vi "Close.vi"(8 "error in (no error)":errorcluster, 11 "SS P100 Settings":T1) -> (0 "error out":errorcluster, 3 "SS P100 Settings":T1)   [LabVIEW 2018, in "Sonic Systems P100.lvlib"]
uses:
  Sonic Systems P100.lvlib
  Sonic Systems P100 Settings.ctl
  support/Support Library.lvlib
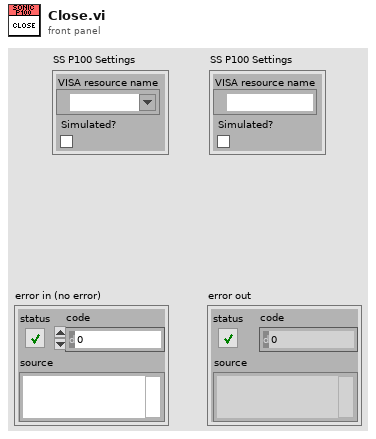
[diagram p1: front panel]
types:
  T1 = typedef "Sonic Systems P100.lvlib/Sonic Systems P100 Settings.ctl" = cluster{"VISA resource name":refnum<visa-resource-name>, "Simulated?":bool}
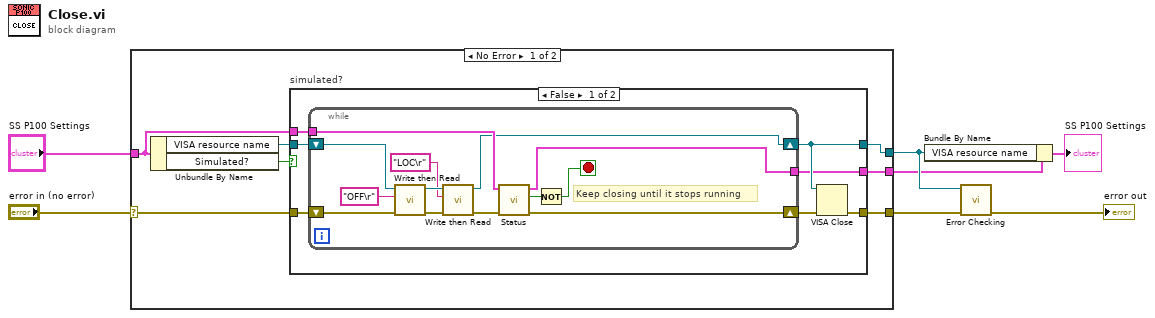
[diagram p0: block diagram]
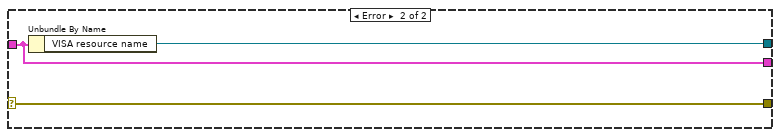
[diagram p3: hidden frame]
diagram:
  n1 = case shown="No Error" "error in (no error)" {
    selector: "error in (no error)" -> [w12 w40]
    tunnel: [w13 w40] -> w6
    tunnel: "SS P100 Settings" -> [w9 w38]
    tunnel: [w10 w39] -> w4
    tunnel: [w8 w38] -> w3
    frame No Error {
      n2 = Unbundle By Name(w9) -> ("VISA resource name"=w11:refnum<visa-resource-name>, "Simulated?"=w14:bool)
      n3 = case "simulated?" shown="False" w14 {
        tunnel: [w19 w37] -> w13
        tunnel: w11 -> [w18 w36]
        tunnel: w12 -> [w21 w37]
        tunnel: [w17 w36] -> w10
        tunnel: w9 -> [w16 w35]
        tunnel: [w15 w35] -> w8
        frame False {
          n4 = while {
            shift-right: [w34] -> w20
            shift-left: w21 -> [w27]
            shift-right: [w23] -> w17
            shift-left: w18 -> [w28]
            tunnel: w16 -> [w30]
            tunnel: [w31] -> w15
            stop <- w33 stop-if-true
            # "Keep closing until it stops running"
            n5 = call "Write then Read.vi"("error in"=w27, "write buffer"="OFF\r" ("string"), "VISA resource name in"=w28) -> ("error out"=w26:errorcluster, "VISA resource name out"=w25:refnum<visa-resource-name>)  [unwired: 6 in, 1 out]
            n6 = call "Write then Read.vi"("error in"=w26, "write buffer"="LOC\r" ("string"), "VISA resource name in"=w25) -> ("error out"=w22:errorcluster, "VISA resource name out"=w23:refnum<visa-resource-name>)  [unwired: 6 in, 1 out]
            n7 = call "Status.vi"("error in (no error)"=w22, "SS P100 Settings In"=w30) -> ("error out"=w34:errorcluster, "Running"=w32:bool, "SS P100 Settings Out"=w31:T1)  [unwired: 4 in, 3 out]
            n8 = Not(x=w32) -> (.not. x?=w33:bool)
          }
          n9 = VISA Close(VISA resource name=w17, error in (no error)=w20) -> (error out=w19:errorcluster)
        }
        frame True {
        }
      }
    }
    frame Error {
      n10 = Unbundle By Name(w38) -> ("VISA resource name"=w39:refnum<visa-resource-name>)
    }
  }
  n11 = Bundle By Name(cluster=w3, "VISA resource name"=w4) -> (→"SS P100 Settings":T1)
  n12 = call "Error Checking.vi"("error in (no error)"=w6, "VISA resource name"=w4) -> ("error out"=→"error out":errorcluster)  [unwired: 7 in, 2 out]
